vi "(SubVI)Ring Itme to Voltage Range.vi"(10 "error in (no error)":errorcluster caption="에러 입력(에러 없음)", 11 "Voltage Range Ring Ref (U8)":refnum<vi>) -> (2 "error out":errorcluster caption="에러 출력", 3 "Voltage Range":dbl)   [LabVIEW 2020]
uses:
  4e0ab527-850a-49fc-8c7e-9f09aaf091c0.vi
  <vilib>/Comparison/Equal/Equal Functor/Equal Functor.lvclass
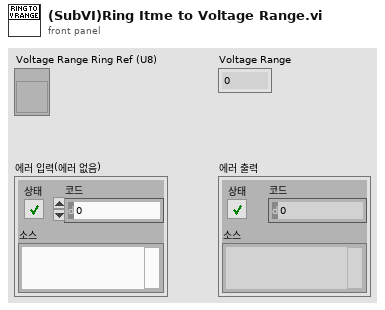
[diagram p1: front panel]
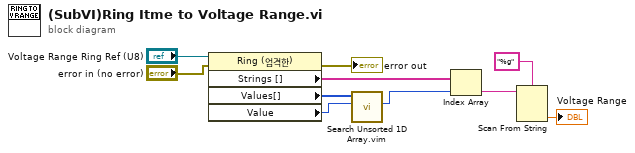
[diagram p0: block diagram]
diagram:
  n1 = property class="Ring (엄격한)"(reference="Voltage Range Ring Ref (U8)", error in="error in (no error)") -> (error out=→"error out":errorcluster, "Strings []"=w2:string[], "Values[]"=w4:u8[], "Value"=w3:u8)  [unwired: 1 out]
  n2 = call "Search Unsorted 1D Array.vim"("element"=w3, "unsorted 1D array"=w4) -> ("index of element"=w1:i32)  [unwired: 9 in]
  n3 = Index Array(array=w2, index=w1) -> (element=w10:string)
  n4 = Scan From String(format string="%g" ("포맷 문자열"), input string=w10) -> (output 1=→"Voltage Range":dbl)  [unwired: 3 in, 3 out]
